vi "Demosaic Image.vi"(0 "grey":u16, 1 "info":T1, 5 "red":u16, 7 "green":u16, 9 "blue":u16) -> (3 "info out":T1, 4 "grey out":u16, 6 "red out":u16, 8 "green out":u16, 10 "blue out":u16, 14 "function return":u32)   [LabVIEW 2018, in "AndorSDK.lvlib"]
doc: "EXPNETTYPE unsigned int WINAPI DemosaicImage(WORD * grey, WORD * red, WORD * green, WORD * blue, ColorDemosaicInfo * info);"
uses:
  AndorSDK.lvlib
  ATMCD32D.dll
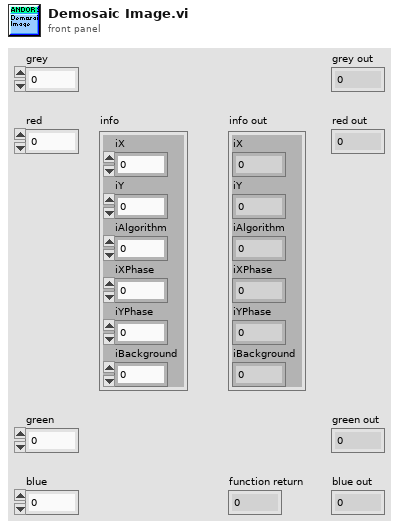
[diagram p1: front panel]
types:
  T1 = cluster{"iX":i32, "iY":i32, "iAlgorithm":i32, "iXPhase":i32, "iYPhase":i32, "iBackground":i32}
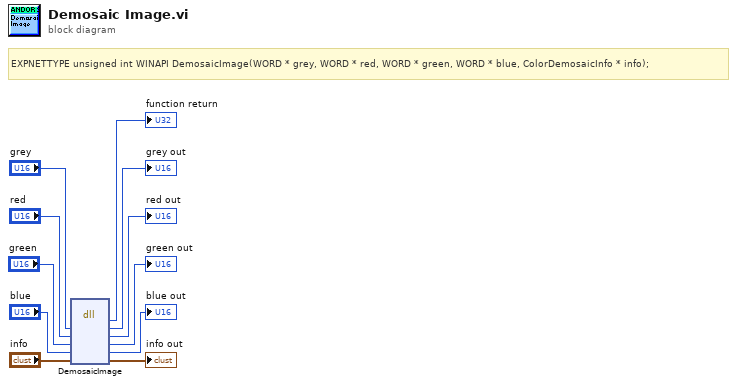
[diagram p0: block diagram]
diagram:
  # "EXPNETTYPE unsigned int WINAPI DemosaicImage(WORD * grey, WORD * red, WORD * green, WORD * blue, ColorDemosaicInfo * info);"
  n1 = dll-call lib="PTH2babs E\nPersönliches02 - Arbeit03-HiwijobsLabviewCodelibANDOR\tAndor SDK\nATMCD32D.*" fn="DemosaicImage"("grey"="grey", "red"="red", "green"="green", "blue"="blue", "info"="info") -> (→"function return":u32, "grey"=→"grey out":u16, "red"=→"red out":u16, "green"=→"green out":u16, "blue"=→"blue out":u16, "info"=→"info out":T1)  [unwired: 3 in, 2 out]
